vi "illegal characters.vi"() -> (1 "Array of illegal characters":string[](array[string])=["(", ")", "-", ". ", "\\", "/", ">", "<", "*", "\"", "£", "$", "+", "=", "&", "!", "\"", "£", "$", "%", "^", "[", "]", "{", "}", "`", "¬"])   [LabVIEW 2017]
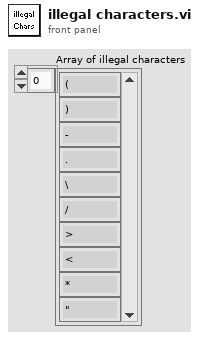
[diagram p1: front panel]
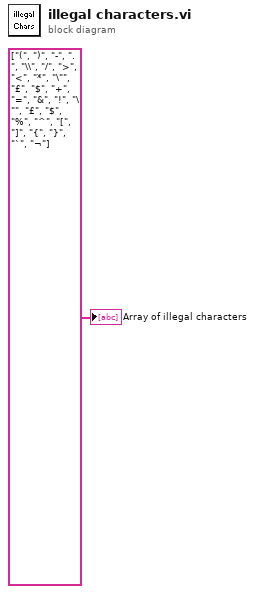
[diagram p0: block diagram]
diagram:
  "Array of illegal characters" <- string[] ["(", ")", "-", ". ", "\\", "/", ">", "<", "*", "\"", "£", "$", "+", "=", "&", "!", "\"", "£", "$", "%", "^", "[", "]", "{", "}", "`", "¬"] ("Array of illegal characters or whole words")
